vi "SIM Is Discrete Tick.vi"(6 "min step size":dbl, 8 "initial time":dbl, 9 "time (ticks)":i32, 10 "tick period (sec)":dbl, 11 "simulation time":dbl) -> (3 "Discrete Tick?":bool)   [LabVIEW 2017]
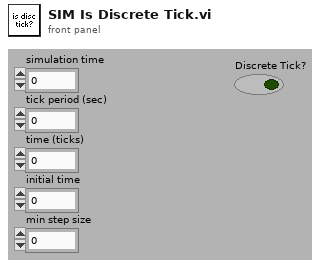
[diagram p1: front panel]
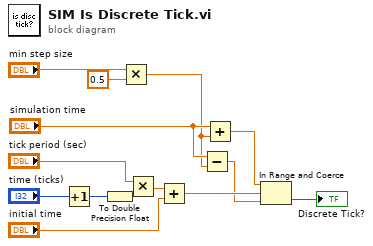
[diagram p0: block diagram]
diagram:
  n1 = Increment(x="time (ticks)") -> (x+1=w10:i32)
  n2 = To Double Precision Float(number=w10) -> (double precision float=w1:dbl)
  n3 = Multiply(x="min step size", y=0.5) -> (x*y=w5:dbl)
  n4 = Multiply(x="tick period (sec)", y=w1) -> (x*y=w13:dbl)
  n5 = Add(x=w13, y="initial time") -> (x+y=w7:dbl)
  n6 = Subtract(x="simulation time", y=w5) -> (x-y=w3:dbl)
  n7 = Add(x="simulation time", y=w5) -> (x+y=w4:dbl)
  n8 = In Range and Coerce(upper limit=w4, x=w7, lower limit=w3) -> (In Range?=→"Discrete Tick?":bool)  [unwired: 1 out]
